vi "Update Errors and Info.vi"(8 "error in (no error)":errorcluster, 9 "Get All Info":bool, 10 "Get All Errors":bool, 11 "CIF_UI in":refnum<class "CIF_Manager_UI.lvclass">) -> (0 "error out":errorcluster, 1 "Info":string, 2 "Error Count":i32, 3 "CIF_UI out":refnum<class "CIF_Manager_UI.lvclass">)   [LabVIEW 2021, in "CIF_Manager_UI.lvclass"]
uses:
  CIF_Manager_UI.lvclass
  C:/Program Files/National Instruments/LabVIEW 2021/vi.lib/CIF Foundation/CIF Core/CIFUI/CIF_UI.lvclass
  CIF_Manager_UI.lvclass/CIF_Manager_UI.ctl
  <vilib>/CIF Foundation/CIF Core/CIFUI/CIF_UI.lvclass/CIF_UI.ctl
  <vilib>/CIF Foundation/CIF Core/CIFUI/Accessors/Read Manager gRPC ID.vi
  <vilib>/CIF Foundation/CIF Core/CIFUI/Accessors/Read Manager Connection.vi
  <vilib>/CIF Foundation/CIF Core/CIFPluginManager/gRPC/CIF_Manager_Client_Wrapper/CIFManagerClientWrapper.lvlib
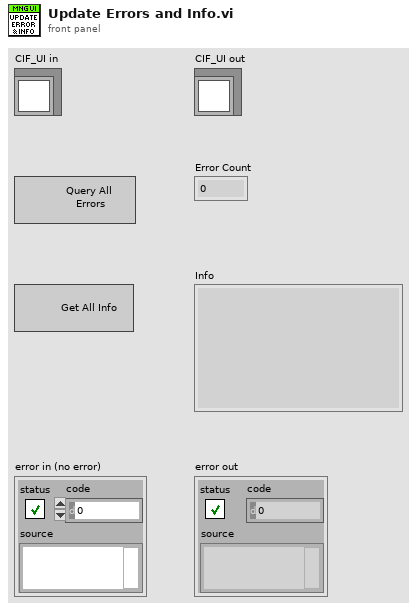
[diagram p1: front panel]
types:
  T1 = typedef "grpc-lvsupport-release.lvlib/grpcId.ctl" = u64
  T2 = typedef "CIF_Manager_client.lvlib/cif_manager_ErrorInfo.ctl" = cluster{"error_status":bool, "error_code":i32, "plugin":string, "time":string, "message":string, "location":string}
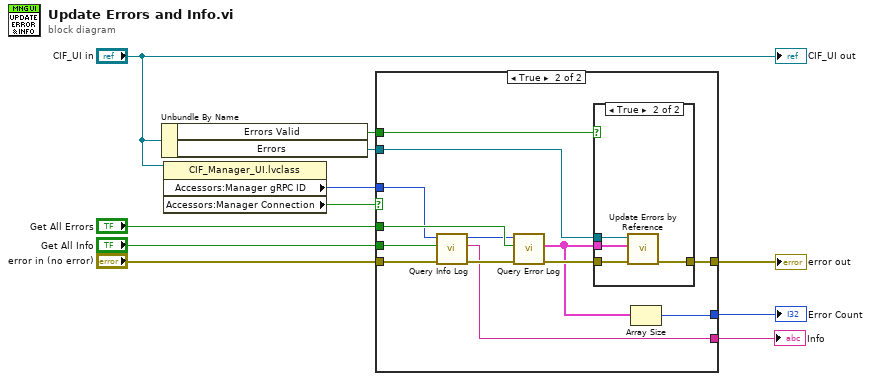
[diagram p0: block diagram]
diagram:
  n1 = Unbundle By Name("CIF_UI in") -> ("Errors Valid"=w4:bool, "Errors"=w9:refnum<vi>)
  n2 = property class="CIF_Manager_UI.lvclass"(reference="CIF_UI in") -> ("Accessors:Manager gRPC ID"=w1:T1, "Accessors:Manager Connection"=w2:bool)  [unwired: 1 in, 2 out]
  n3 = case shown="True" w2 {
    tunnel: "Get All Errors" -> [_ w24]
    tunnel: "Get All Info" -> [_ w23]
    tunnel: w9 -> [_ w21]
    tunnel: [w12 w18] -> w8
    tunnel: [_ w17] -> w7
    tunnel: [_ w16] -> w6
    tunnel: w1 -> [_ w15]
    tunnel: "error in (no error)" -> [w12 w14]
    tunnel: w4 -> [_ w13]
    frame False {
    }
    frame True {
      n4 = call <vilib>:"Query Info Log.vi"("error in"=w14, "query_all"=w23, "gRPC ID in"=w15) -> ("error out"=w19:errorcluster, "Info"=w16:string, "gRPC ID out"=w20:T1)  [unwired: 6 in]
      n5 = call <vilib>:"Query Error Log.vi"("error in"=w19, "query_all"=w24, "gRPC ID in"=w20) -> ("error out"=w25:errorcluster, "error_info"=w22:T2[])  [unwired: 6 in, 1 out]
      n6 = case shown="True" w13 {
        tunnel: w25 -> [w26 w30]
        tunnel: w22 -> [_ w29]
        tunnel: w21 -> [_ w28]
        tunnel: [w26 w27] -> w18
        frame False {
        }
        frame True {
          n7 = call "Update Errors by Reference.vi"("error in (no error)"=w30, "error_info"=w29, "Error MCLB reference in"=w28) -> ("error out"=w27:errorcluster)  [unwired: 7 in, 1 out]
        }
      }
      n8 = Array Size(array=w22) -> (size(s)=w17:i32)
    }
  }
  "error out" <- w8
  "Error Count" <- w7
  "Info" <- w6
  "CIF_UI out" <- "CIF_UI in"
